vi "Shooter Immediate Wrapper.vi"() -> ()   [LabVIEW 2019]
panel:
  in  "Hood Setpoint":dbl
  in  "Flywheel Setpoint":dbl
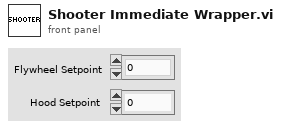
[diagram p1: front panel]
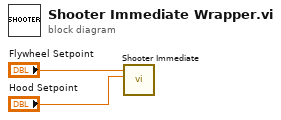
[diagram p0: block diagram]
diagram:
  n1 = call "Shooter Immediate.vi"("Hood Setpoint"="Hood Setpoint", "Flywheel Setpoint"="Flywheel Setpoint") -> ()  [unwired: 9 in, 1 out]
